vi "Luis.vi"() -> ()   [LabVIEW 2017]
uses:
  <vilib>/Motion/Express/_s/nimc.fb.read.readExecutionData.axis.vi
  <vilib>/Motion/Express/_s/nimc.fb.straightLineMove.startStraightLineMove.axis.modeAbsolute.0.vi
  <vilib>/Motion/BlockNode/FB.NIMotion.xnode
panel:
  in  "Array":T1(array[cluster])=[{"Enum"=enum."lineal", "Numeric"=0.0}, {"Enum"=enum."lineal", "Numeric"=0.0}, {"Enum"=enum."lineal", "Numeric"=0.0}, {"Enum"=enum."lineal", "Numeric"=0.0}, {"Enum"=enum."lineal", "Numeric"=0.0}, {"Enum"=enum."lineal", "Numeric"=0.0}, {"Enum"=enum."lineal", "Numeric"=0.0}, {"Enum"=enum."lineal", "Numeric"=0.0}, {"Enum"=enum."lineal", "Numeric"=0.0}, {"Enum"=enum."lineal", "Numeric"=0.0}, {"Enum"=enum."lineal", "Numeric"=0.0}, {"Enum"=enum."lineal", "Numeric"=0.0}, {"Enum"=enum."lineal", "Numeric"=0.0}, {"Enum"=enum."lineal", "Numeric"=0.0}, {"Enum"=enum."lineal", "Numeric"=0.0}, {"Enum"=enum."lineal", "Numeric"=0.0}, {"Enum"=enum."lineal", "Numeric"=0.0}, {"Enum"=enum."lineal", "Numeric"=0.0}, {"Enum"=enum."lineal", "Numeric"=0.0}, {"Enum"=enum."lineal", "Numeric"=0.0}, {"Enum"=enum."lineal", "Numeric"=0.0}, {"Enum"=enum."lineal", "Numeric"=0.0}, {"Enum"=enum."lineal", "Numeric"=0.0}, {"Enum"=enum."lineal", "Numeric"=0.0}, {"Enum"=enum."lineal", "Numeric"=0.0}]
  in  "Stop Button":bool
  out "Slide 2":dbl(slide) scale=0.0..16.0
  out "Slide":dbl(slide)=-0.0 scale=0.0..6.0
  out "XY Graph":cluster{dbl[], dbl[]}(graph)
  # "*"
  # "k"
  # "*"
  # "."
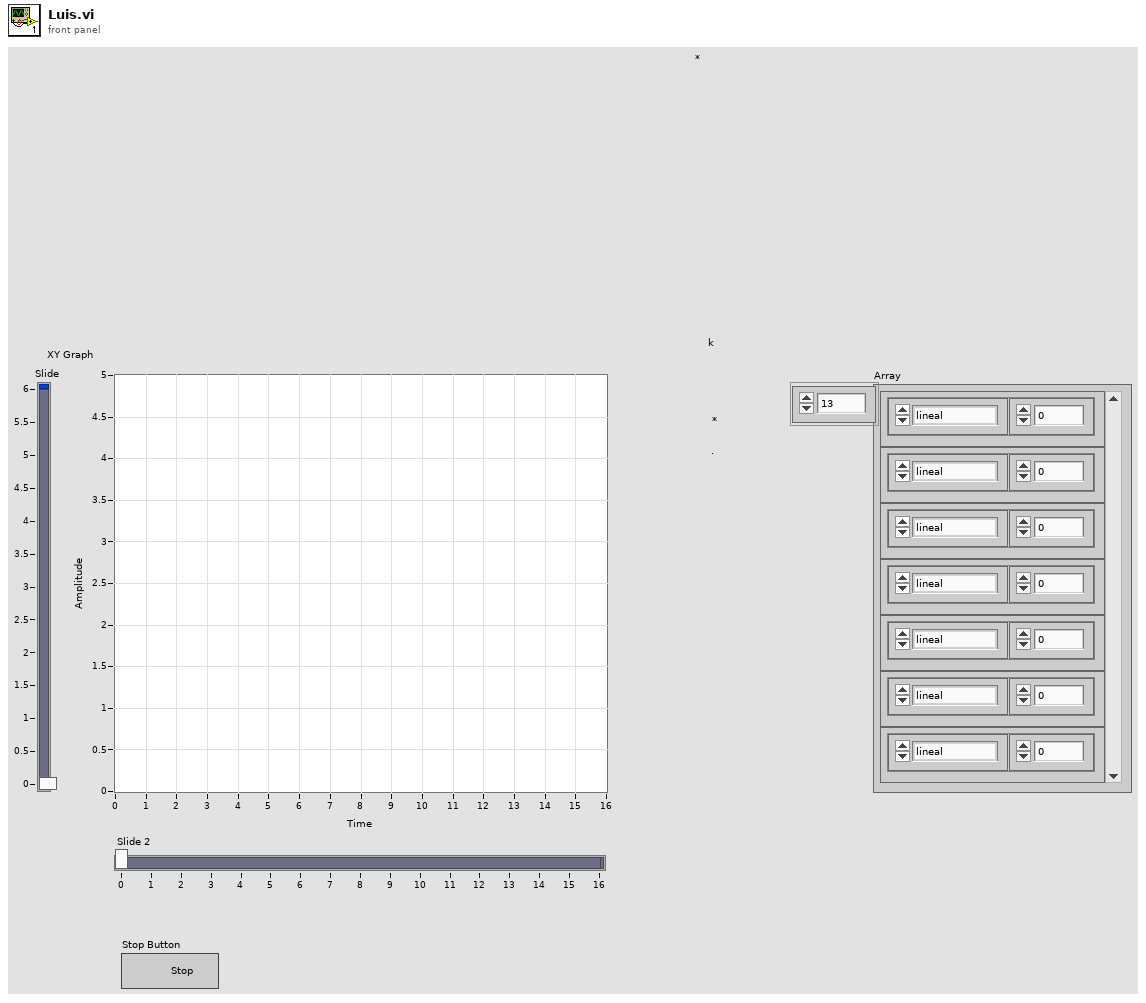
[diagram p1: front panel]
types:
  T1 = cluster{"Enum":enum16{"Circular", "lineal"}, "Numeric":dbl}[]
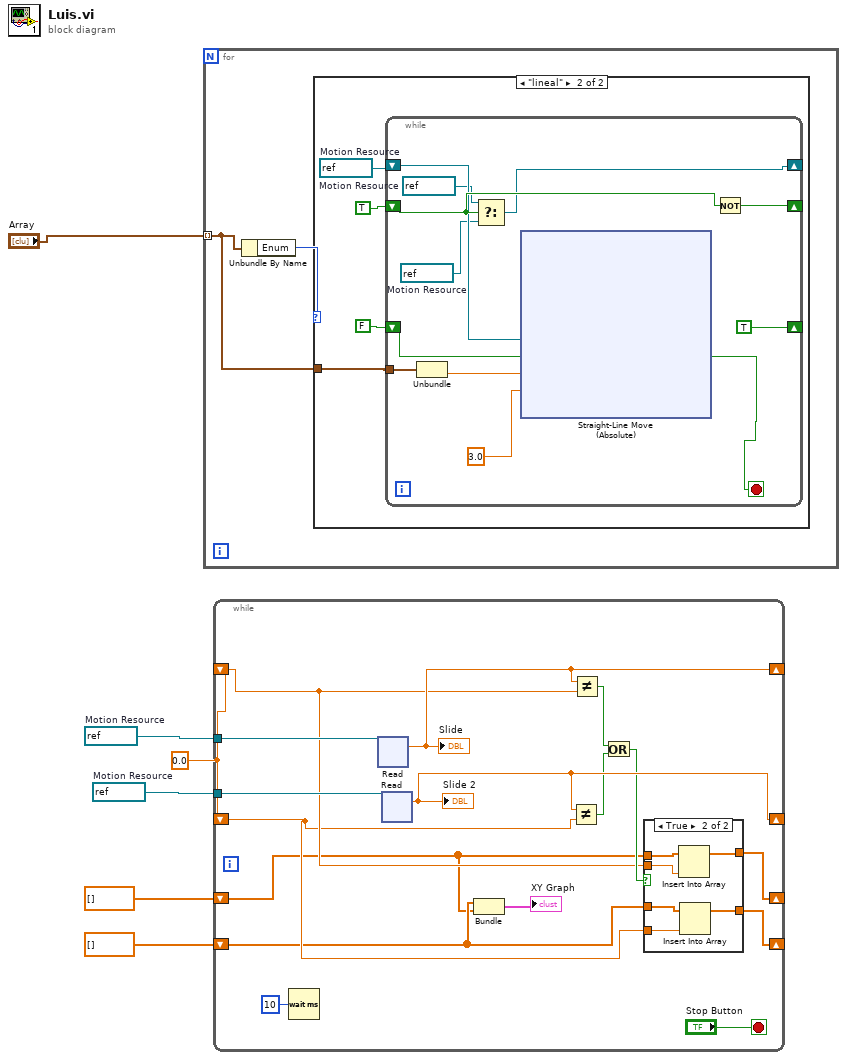
[diagram p0: block diagram]
diagram:
  w4 = 0.0 ("position")
  w5 = refnum<k21> "Eje X"  # Motion Resource
  w6 = refnum<k21> "Eje Y"  # Motion Resource
  n1 = for {
    tunnel: "Array" -> [w7] mode=indexing
    n2 = Unbundle By Name(w7) -> ("Enum"=w8:enum16{"Circular", "lineal"})
    n3 = case shown="\"lineal\"" w8 {
      tunnel: w7 -> [_ w12]
      frame "Circular", Default {
      }
      frame "lineal" {
        w9 = refnum<k21> "Eje X"  # Motion Resource
        n4 = while {
          tunnel: w12 -> [w20]
          shift-right: [TRUE] -> _
          shift-left: FALSE -> [w22]
          shift-right: [w18] -> _
          shift-left: TRUE -> [w17]
          shift-right: [w13] -> _
          shift-left: w9 -> [w16]
          stop <- w23 stop-if-true
          w14 = refnum<k21> "Eje X"  # Motion Resource
          w15 = refnum<k21> "Eje Y"  # Motion Resource
          n5 = Unbundle(w20) -> ("Numeric"=w19:dbl)  [unwired: 1 out]
          n6 = Select(t=w14, s=w17, f=w15) -> (s? t:f=w13:refnum<k21>)
          n7 = xnode "Straight-Line Move\n(Absolute)"("resource"=w16, "execute"=w22, "position"=w19, "velocity"=3.0) -> ("done"=w23:bool)  [unwired: 2 in, 2 out]
          n8 = Not(x=w17) -> (.not. x?=w18:bool)
        }
      }
    }
  }
  n9 = while {
    tunnel: w6 -> [w57]
    tunnel: w5 -> [w56]
    shift-right: [w54] -> _
    shift-left: w4 -> [w47]
    shift-right: [w55] -> _
    shift-left: w4 -> [w48]
    shift-right: [w49] -> _
    shift-left: dbl[] [] -> [w44]
    shift-right: [w50] -> _
    shift-left: dbl[] [] -> [w43]
    stop <- "Stop Button" stop-if-true
    n10 = Wait (ms)(milliseconds to wait=u32 10) -> ()  [unwired: 1 out]
    n11 = xnode "Read"("resource"=w57) -> ("position"=w55:dbl)  [unwired: 2 in, 7 out]
    "Slide" <- w55
    n12 = xnode "Read"("resource"=w56) -> ("position"=w54:dbl)  [unwired: 2 in, 7 out]
    "Slide 2" <- w54
    n13 = Bundle(w44, w43) -> (→"XY Graph":cluster{dbl[], dbl[]})  [unwired: 1 in]
    n14 = Not Equal?(x=w54, y=w47) -> (x != y?=w53:bool)
    n15 = Not Equal?(x=w55, y=w48) -> (x != y?=w52:bool)
    n16 = Or(x=w52, y=w53) -> (x .or. y?=w51:bool)
    n17 = case shown="True" w51 {
      tunnel: w43 -> [w59 w65]
      tunnel: [w59 w64] -> w50
      tunnel: w44 -> [w58 w63]
      tunnel: [w58 w62] -> w49
      tunnel: w48 -> [_ w61]
      tunnel: w47 -> [_ w60]
      frame False {
      }
      frame True {
        n18 = Insert Into Array(array=w65, new element=w61) -> (w64:dbl[])  [unwired: 1 in]
        n19 = Insert Into Array(array=w63, new element=w60) -> (w62:dbl[])  [unwired: 1 in]
      }
    }
  }
